vi "Calculate High G sum.vi"(1 "Z axis":dbl[](array[numeric]), 2 "Y axis":dbl[](array[numeric]), 3 "X axis":dbl[](array[numeric])) -> (0 "Sum":dbl[](array[numeric]))   [LabVIEW 2011]
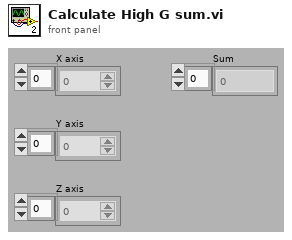
[diagram p1: front panel]
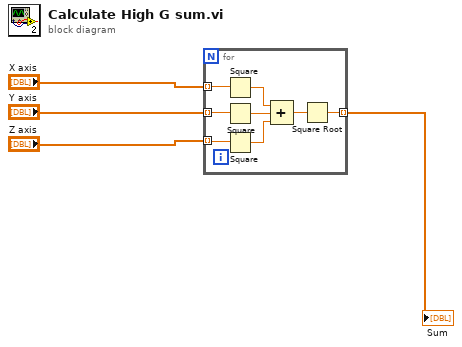
[diagram p0: block diagram]
diagram:
  n1 = for {
    tunnel: "X axis" -> [w12] mode=indexing
    tunnel: "Y axis" -> [w11] mode=indexing
    tunnel: "Z axis" -> [w10] mode=indexing
    tunnel: [w5] -> w4 mode=indexing
    n2 = Square(x=w12) -> (x^2=w8:dbl)
    n3 = Square(x=w11) -> (x^2=w9:dbl)
    n4 = Square(x=w10) -> (x^2=w7:dbl)
    n5 = Compound Arithmetic op=ADD(w8, w9, w7) -> (w6:dbl)
    n6 = Square Root(x=w6) -> (sqrt(x)=w5:dbl)
  }
  "Sum" <- w4
